vi "Read Status.vi"(8 "error in (no error)":errorcluster, 11 "Channel in":refnum<data-value>) -> (0 "error out":errorcluster, 2 "Channel Status":T1, 3 "Channel out":refnum<data-value>)   [LabVIEW 2020, in "G-Audio.lvlib" / "Channel.lvclass"]
uses:
  Channel.lvclass
  Controls/Channel Status.ctl
  Controls/Channel State.ctl
  Channel.lvclass/Channel.ctl
  d1584b72-7993-414d-864f-32a53ed84d25.vi
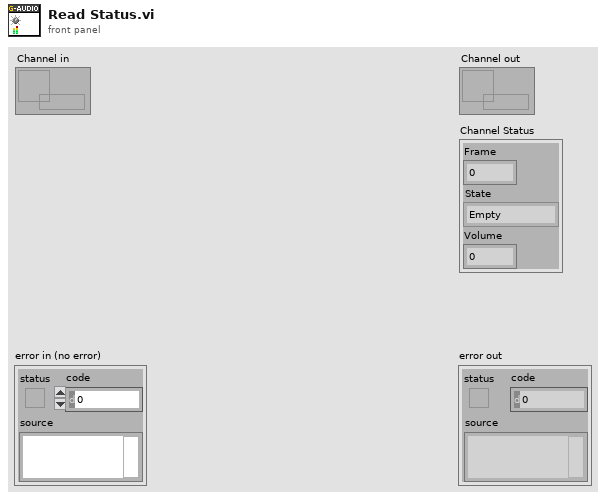
[diagram p1: front panel]
types:
  T1 = typedef "G-Audio.lvlib/Channel.lvclass/Channel Status.ctl" = cluster{"Frame":u64, "State":T2, "Volume":sgl}
  T2 = typedef "G-Audio.lvlib/Channel.lvclass/Channel State.ctl" = enum16{"Empty", "Loading", "Stopped", "Paused", "Playing", "Retrigger"}
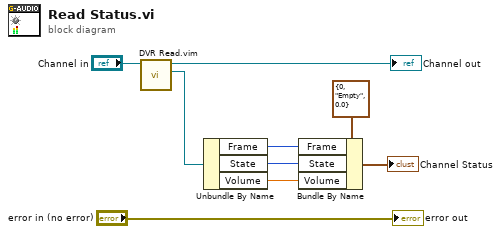
[diagram p0: block diagram]
diagram:
  n1 = call "DVR Read.vim"("DVR In"="Channel in") -> ("Data"=w2:refnum<class "Channel.lvclass">, "DVR Out"=→"Channel out":refnum<data-value>)  [unwired: 9 in]
  n2 = Unbundle By Name(w2) -> ("Frame"=w8:u64, "State"=w7:T2, "Volume"=w6:sgl)
  n3 = Bundle By Name(cluster=T1 {"Frame"=0, "State"=enum."Empty", "Volume"=0.0} ("Channel Status"), "Frame"=w8, "State"=w7, "Volume"=w6) -> (→"Channel Status":T1)
  "error out" <- "error in (no error)"
